vi "W vs Z Lens & free space array.vi"(4 "lens focal length":dbl=-250.0 format="%.3f", 6 "FWHM(T)?":bool, 7 "Wavelength":dbl=0.0007 format="%.6f", 8 "Q in":cdb format="%.2f", 9 "N steps":i32=1, 10 "z stop":dbl=1000.0 format="%.2f", 11 "z start":dbl format="%.2f") -> (0 "Q out":cdb format="%.2f", 1 "Q Array":cxt[](array[numeric]) format="%.2f", 2 "w/FWHM Array":dbl[](array[numeric]) format="%.2f", 3 "Z Array":dbl[](array[numeric]) format="%.2f", 5 "W/FWHM vs Z":cluster{dbl[], dbl[]}(graph))   [LabVIEW 2016]
panel:
  out "sig min z":dbl format="%.2f"
  out "min signa w":dbl format="%.8f"
  out "Q start":cdb format="%.4f"
  in  "beam radius(w)":dbl=0.002 format="%.3f"
  in  "Radius of Curvature":dbl=inf format="%.2f"
  out "z step":dbl=1.0 format="%.3f"
  # "This consolidates a lens followed by a free space region"
  # "All values are entered in mm"
  # "w is the 1/e field radius"
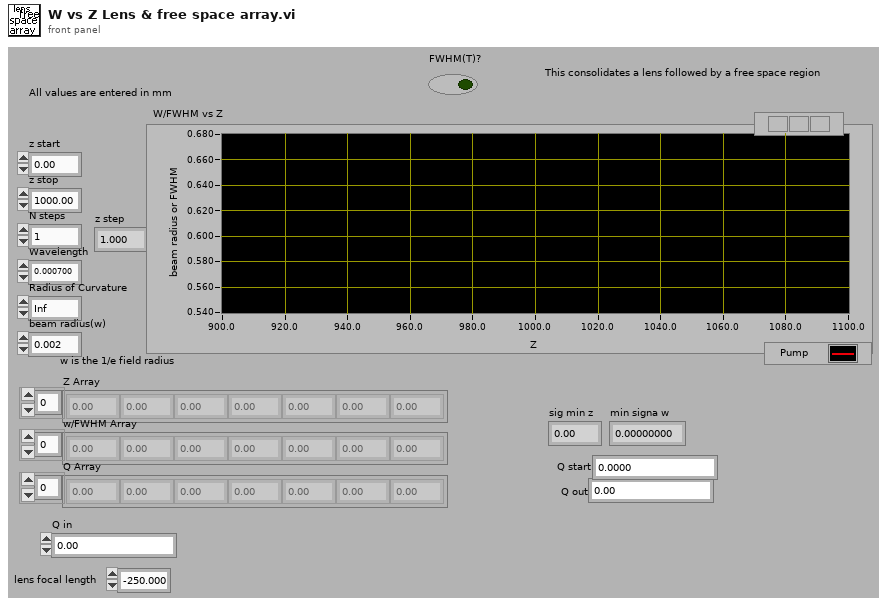
[diagram p1: front panel]
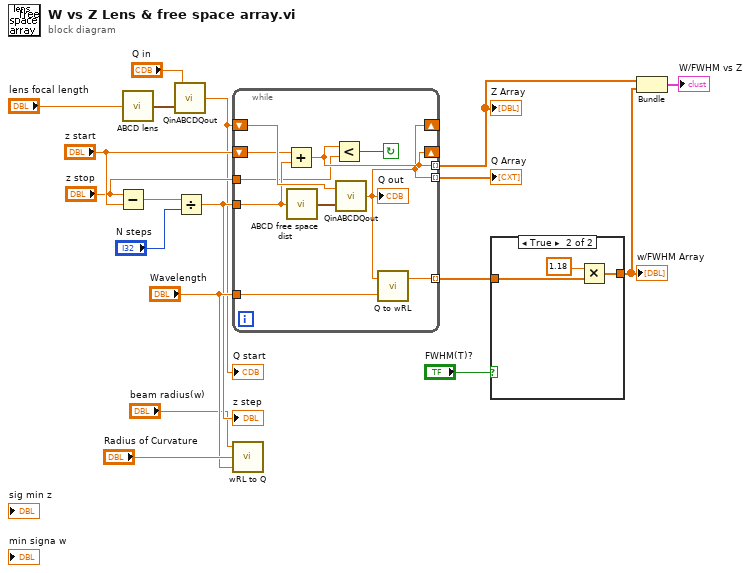
[diagram p0: block diagram]
diagram:
  n1 = Subtract(x="z stop", y="z start") -> (x-y=w14:dbl)
  n2 = call "ABCD lens.vi"("Focal length"="lens focal length") -> ("ABCD"=w4:cluster{"A":dbl, "B":dbl, "C":dbl, "D":dbl})
  n3 = call "QinABCDQout.vi"("ABCD"=w4, "Q in"="Q in") -> ("Q out"=w2:cdb)
  "Q start" <- w2
  n4 = Divide(x=w14, y="N steps") -> (x/y=w12:dbl)
  "z step" <- w12
  n5 = while {
    shift-right: [w24] -> _
    shift-left: "z start" -> [w22]
    tunnel: w12 -> [w23]
    shift-right: [w19] -> _
    shift-left: w2 -> [w26]
    tunnel: "Wavelength" -> [w25]
    tunnel: [w20] -> w6 mode=indexing
    tunnel: [w24] -> w10 mode=indexing
    tunnel: "z stop" -> [w21]
    tunnel: [w19] -> w9 mode=indexing
    stop <- w28 continue-if-true
    n6 = Add(x=w22, y=w23) -> (x+y=w24:dbl)
    n7 = call "ABCD free space dist.vi"("Dist"=w23) -> ("ABCD"=w27:cluster{"A":dbl, "B":dbl, "C":dbl, "D":dbl})
    n8 = Less?(x=w24, y=w21) -> (x < y?=w28:bool)
    n9 = call "QinABCDQout.vi"("ABCD"=w27, "Q in"=w26) -> ("Q out"=w19:cdb)
    "Q out" <- w19
    n10 = call "Q to wRL.vi"("Wavelength"=w25, "Q"=w19) -> ("beam radius(w)"=w20:dbl)  [unwired: 1 out]
  }
  "Z Array" <- w10
  "Q Array" <- w9
  n11 = call "wRL to Q.vi"("Wavelength"="Wavelength", "Radius of Curvature"="Radius of Curvature", "beam radius(w)"="beam radius(w)") -> ()  [unwired: 1 out]
  n12 = case shown="True" "FWHM(T)?" {
    tunnel: w6 -> [w29 w31]
    tunnel: [w29 w30] -> w5
    frame False {
    }
    frame True {
      n13 = Multiply(x=1.18, y=w31) -> (x*y=w30:dbl[])
    }
  }
  "w/FWHM Array" <- w5
  n14 = Bundle(w10, w5) -> (→"W/FWHM vs Z":cluster{dbl[], dbl[]})  [unwired: 1 in]
